vi "getTimeLength.vi"(8 "error in (no error)":errorcluster, 10 "Path":path, 11 "playFileAction":refnum<class "playFileAction.lvclass">) -> (0 "error out":errorcluster, 2 "timeLength":dbl, 3 "playFileAction out":refnum<class "playFileAction.lvclass">)   [LabVIEW 2011, in "Views.lvlib" / "ScriptEditor.lvlib" / "playFileAction.lvclass"]
uses:
  playFileAction.lvclass
  Tools/Scripting/ScriptingEvent/ScriptEvents/PlayFile/PlayFile.lvclass
  playFileAction.lvclass/playFileAction.ctl
  ActionPanel.lvclass
  Tools/DatabaseHelpers/Database Objects/Channel/Channel.lvclass
  Tools/Scripting/ScriptingEvent/ScriptEvent.lvclass
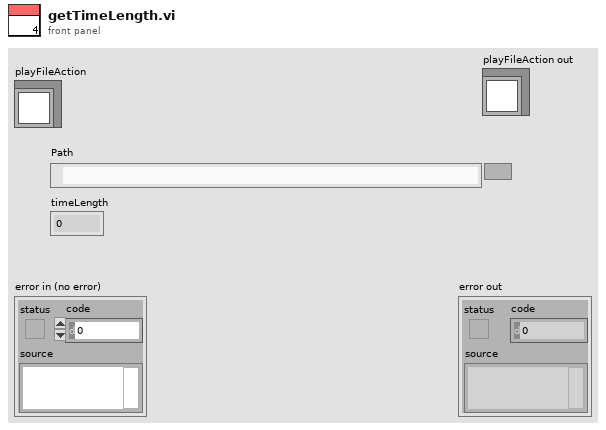
[diagram p1: front panel]
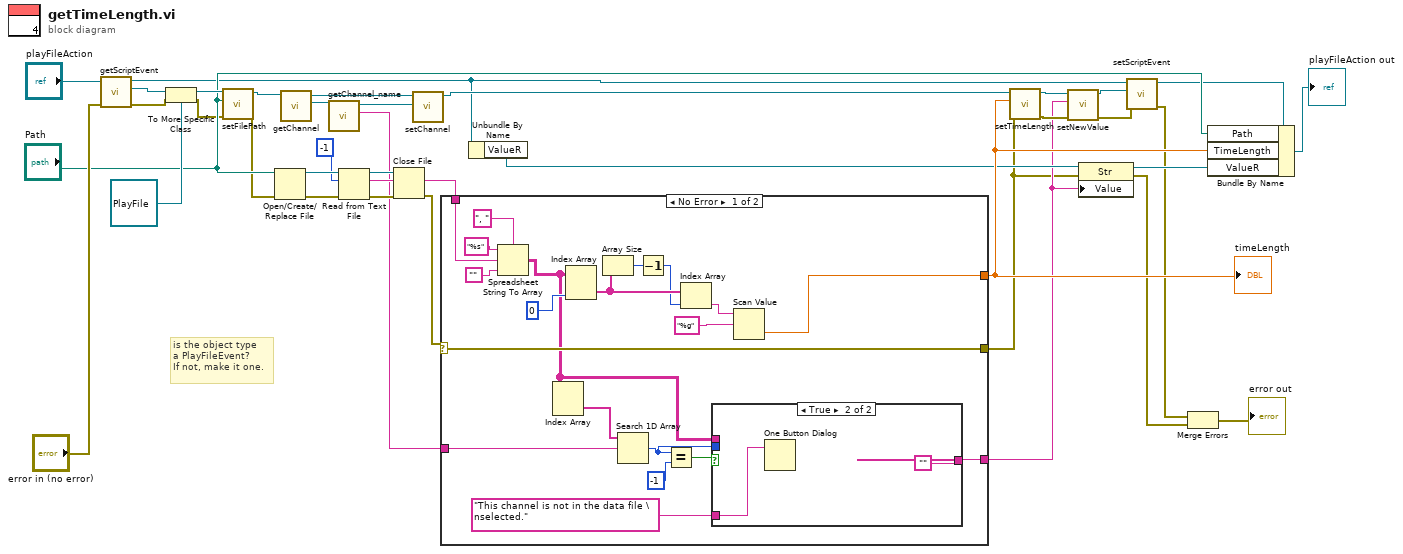
[diagram p0: block diagram]
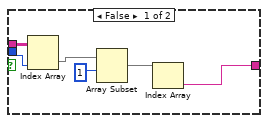
[diagram p2: hidden frame]
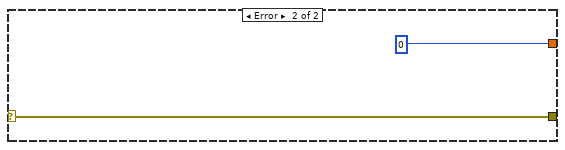
[diagram p3: hidden frame]
diagram:
  # "is the object type\na PlayFileEvent?\nIf not, make it one."
  n1 = call "getScriptEvent.vi"("error in (no error)"="error in (no error)", "ActionPanel.lvclass in"="playFileAction") -> ("error out"=w25:errorcluster, "ScriptEvent.lvclass"=w26:refnum<class "ScriptEvent.lvclass">, "ActionPanel.lvclass out"=w8:refnum<class "playFileAction.lvclass">)  [unwired: 7 in]
  n2 = To More Specific Class(target class=refnum<class "PlayFile.lvclass"> refnum ("Tools.lvlib:Scripting.lvlib:PlayFile.lvclass"), reference=w26, error in=w25) -> (specific class reference=w24:refnum<class "PlayFile.lvclass">, error out=w22:errorcluster)
  n3 = call "setFilePath.vi"("error in (no error)"=w22, "filePath"="Path", "PlayFile in"=w24) -> ("error out"=w21:errorcluster, "PlayFile out"=w17:refnum<class "PlayFile.lvclass">)  [unwired: 7 in]
  n4 = Open/Create/Replace File(file path (use dialog)="Path", error in=w21) -> (refnum out=w37:refnum<file>, error out=w36:errorcluster)  [unwired: 4 in, 1 out]
  n5 = call-dynamic "getChannel.vi"("ScriptEvent.lvclass in"=w17) -> ("Channel.lvclass"=w18:refnum<class "Channel.lvclass">, "ScriptEvent.lvclass out"=w15:refnum<class "PlayFile.lvclass">)  [unwired: 8 in, 1 out]
  n6 = call "getChannel_name.vi"("Channel.lvclass in"=w18) -> ("channel_name"=w16:string, "Channel.lvclass out"=w14:refnum<class "Channel.lvclass">)  [unwired: 8 in, 1 out]
  n7 = Read from Text File(file (use dialog)=w37, count=-1, error in=w36) -> (refnum out=w34:refnum<file>, text=w32:string, error out=w35:errorcluster)  [unwired: 1 in, 1 out]
  n8 = Close File(refnum=w34, error in=w35) -> (error out=w31:errorcluster)  [unwired: 1 out]
  n9 = call-dynamic "setChannel.vi"("Channel.lvclass"=w14, "ScriptEvent.lvclass in"=w15) -> ("ScriptEvent.lvclass out"=w13:refnum<class "PlayFile.lvclass">)  [unwired: 8 in, 1 out]
  n10 = case shown="No Error" w31 {
    selector: w31 -> [w46 w66]
    tunnel: w32 -> [w57 _]
    tunnel: [w47 0] -> w20
    tunnel: [w46 w66] -> w4
    tunnel: w16 -> [w41 _]
    tunnel: [w38 _] -> w5
    frame No Error {
      n11 = Spreadsheet String To Array(delimiter (Tab)=", ", format string="%s", spreadsheet string=w57, array type (2D Dbl)="") -> (array=w40:string[][])
      n12 = Index Array(array=w40) -> (element=w45:string[])  [unwired: 2 in]
      n13 = Index Array(array=w40, index (col)=0 ("disabled index (col)")) -> (element=w51:string[])  [unwired: 1 in]
      n14 = Array Size(array=w51) -> (size(s)=w50:i32)
      n15 = Search 1D Array(1D array=w45, element=w41) -> (index of element=w39:i32)  [unwired: 1 in]
      n16 = Decrement(x=w50) -> (x-1=w48:i32)
      n17 = Equal?(x=w39, y=-1) -> (x = y?=w43:bool)
      n18 = Index Array(array=w51, index=w48) -> (element=w49:string)
      n19 = case shown="True" w43 {
        tunnel: "This channel is not in the data file \nselected." -> [_ w65]
        tunnel: w40 -> [w62 _]
        tunnel: w39 -> [w61 _]
        tunnel: [w58 ""] -> w38
        frame False {
          n20 = Index Array(array=w62, index (col)=w61) -> (element=w63:string[])  [unwired: 1 in]
          n21 = Array Subset(array=w63, index=1) -> (w59:string[])  [unwired: 1 in]
          n22 = Index Array(array=w59) -> (element=w58:string)  [unwired: 1 in]
        }
        frame True {
          n23 = One Button Dialog(message=w65) -> ()  [unwired: 1 in, 1 out]
        }
      }
      n24 = Scan Value(string=w49, format string="%g") -> (value=w47:dbl)  [unwired: 1 in, 1 out]
    }
    frame Error {
    }
  }
  "timeLength" <- w20
  n25 = Unbundle By Name(w8) -> ("ValueR"=w6:refnum<vi>)
  n26 = call "setTimeLength.vi"("error in (no error)"=w4, "timeLength"=w20, "PlayFile in"=w13) -> ("error out"=w10:errorcluster, "PlayFile out"=w12:refnum<class "PlayFile.lvclass">)  [unwired: 7 in]
  n27 = call "setNewValue.vi"("error in (no error)"=w10, "newValue"=w5, "ScriptEvent.lvclass in"=w12) -> ("error out"=w9:errorcluster, "ScriptEvent.lvclass out"=w11:refnum<class "PlayFile.lvclass">)  [unwired: 7 in]
  n28 = property class="Str"(reference=w6, error in=w4, "Value"=w5) -> (reference out=w7:refnum<vi>, error out=w1:errorcluster)
  n29 = call "setScriptEvent.vi"("error in (no error)"=w9, "ScriptEvent.lvclass"=w11, "ActionPanel.lvclass in"=w8) -> ("error out"=w2:errorcluster, "ActionPanel.lvclass out"=w19:refnum<class "playFileAction.lvclass">)  [unwired: 7 in]
  n30 = Merge Errors(w2, w1) -> (→"error out":errorcluster)
  n31 = Bundle By Name(cluster=w19, "Path"="Path", "TimeLength"=w20, "ValueR"=w7) -> (→"playFileAction out":refnum<class "playFileAction.lvclass">)
